vi "Set LVClass Path.vi"(10 "LVClass Path":path, 11 "Identity Writer in":refnum<class "Identity Writer.lvclass">) -> (3 "Identity Writer out":refnum<class "Identity Writer.lvclass">)   [LabVIEW 2013, in "Identity Writer.lvclass"]
uses:
  Identity Writer.lvclass
  Identity Writer.lvclass/Identity Writer.ctl
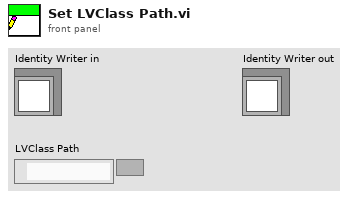
[diagram p1: front panel]
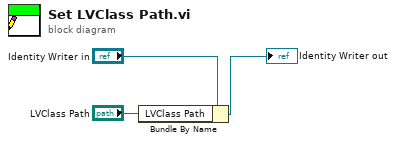
[diagram p0: block diagram]
diagram:
  n1 = Bundle By Name(cluster="Identity Writer in", "LVClass Path"="LVClass Path") -> (→"Identity Writer out":refnum<class "Identity Writer.lvclass">)
